vi "AcquireImage test 2.vi"() -> ()   [LabVIEW 2009]
uses:
  Camera.lvlib
  ImageAnalysis.lvlib
panel:
  out "Walls":T1(array[cluster])
  out "current time":timestamp
  out "Objects bottom cords":T2(array[cluster])
  out "Image":T3(plugin-control)
  out "x-y":u32
  out "Total time":u32
  out "#frames processed":i32
  in  "stop":bool
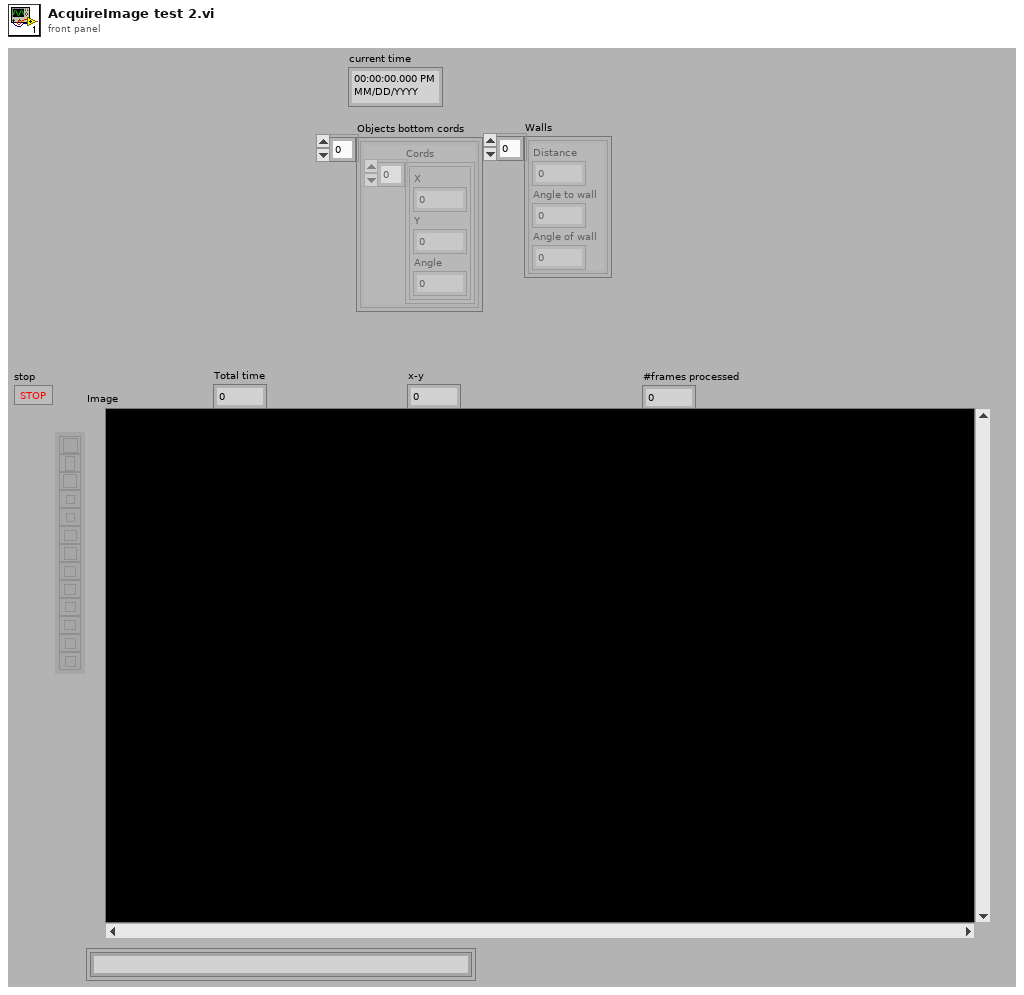
[diagram p1: front panel]
types:
  T1 = cluster{"Distance":dbl, "Angle to wall":dbl, "Angle of wall":dbl}[]
  T2 = cluster{"Cords":cluster{"X":dbl, "Y":dbl, "Angle":dbl}[]}[]
  T3 = typedef "IMAQ Image.ctl" = refnum<image>
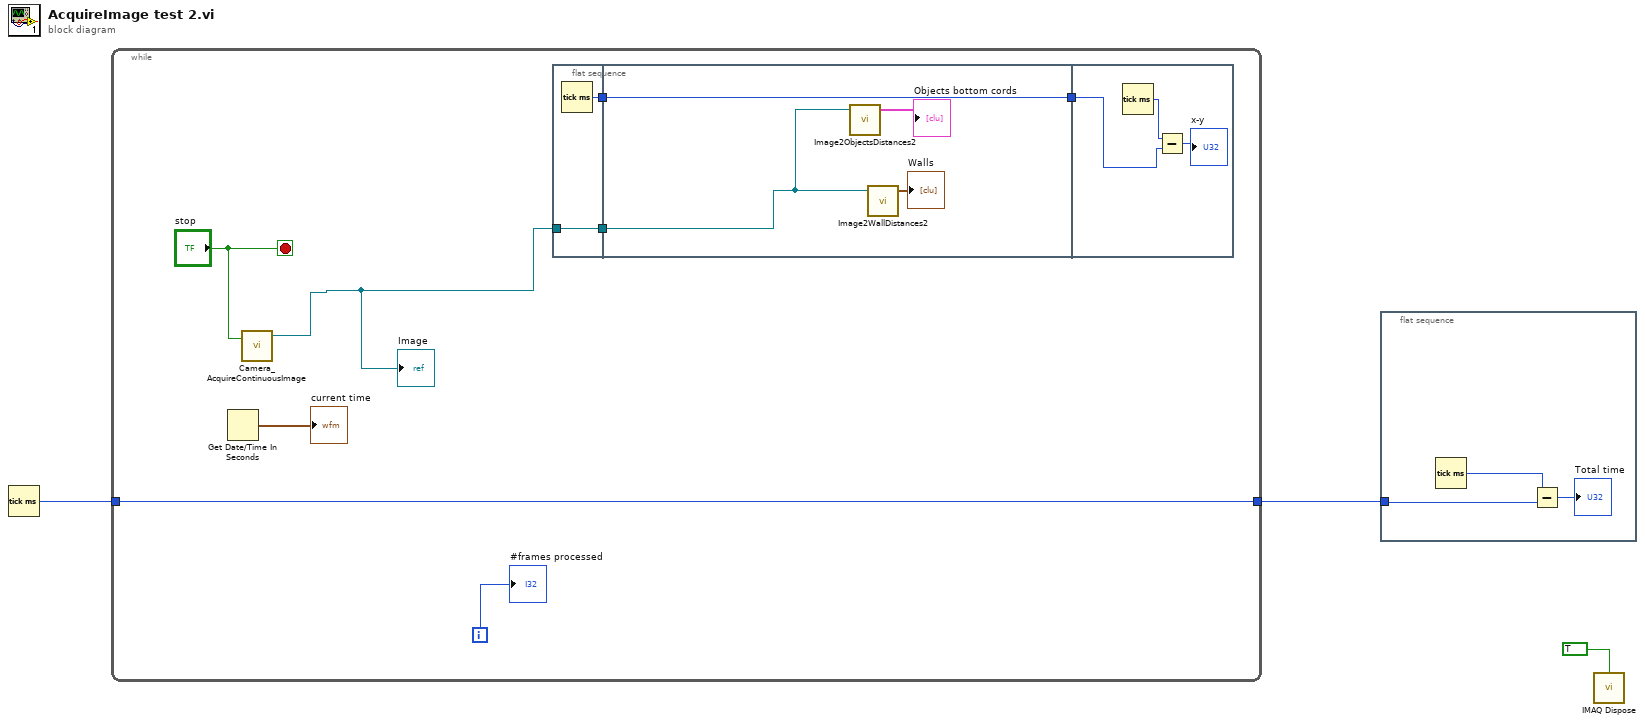
[diagram p0: block diagram]
diagram:
  n1 = Tick Count (ms)() -> (millisecond timer value=w3:u32)
  n2 = while {
    tunnel: w3 -> [w9]
    tunnel: [w9] -> w2
    i -> [w10]
    stop <- "stop" stop-if-true
    n3 = Get Date/Time In Seconds() -> (seconds since 1Jan1904=→"current time":timestamp)
    n4 = call "Camera_AcquireContinuousImage.vi"("Stop (F)"="stop") -> ("Image Out"=w5:T3)  [unwired: 1 in, 2 out]
    "Image" <- w5
    n5 = flat-sequence {
      tunnel: [w13] -> w7
      tunnel: w5 -> [w12]
      tunnel: [w12] -> w6
      tunnel: [w17] -> w8
      tunnel: w7 -> [w17]
      tunnel: w6 -> [w15]
      tunnel: w8 -> [w19]
      frame #0 {
        n6 = Tick Count (ms)() -> (millisecond timer value=w13:u32)
      }
      frame #1 {
        n7 = call "Image2ObjectsDistances2.vi"("Image Src"=w15) -> ("Objects bottom cords"=→"Objects bottom cords":T2)  [unwired: 3 in, 1 out]
        n8 = call "Image2WallDistances2.vi"("Image Src"=w15) -> ("Walls"=→"Walls":T1)  [unwired: 3 in, 1 out]
      }
      frame #2 {
        n9 = Tick Count (ms)() -> (millisecond timer value=w20:u32)
        n10 = Subtract(x=w20, y=w19) -> (x-y=→"x-y":u32)
      }
    }
    "#frames processed" <- w10
  }
  n11 = flat-sequence {
    tunnel: w2 -> [w21]
    frame #0 {
      n12 = Tick Count (ms)() -> (millisecond timer value=w23:u32)
      n13 = Subtract(x=w23, y=w21) -> (x-y=→"Total time":u32)
    }
  }
  n14 = call "IMAQ Dispose"("All Images? (No)"=TRUE) -> ()  [unwired: 5 in, 1 out]
